vi "GRCtoASPICreg.vi"(1 "TM":bool, 2 "AF1":bool, 3 "RC":u8=3 format="%b", 4 "Gain":u8=8 format="%b") -> (0 "aspic1Data":u32[](array[numeric])=[8388739, 8454144, 8519680, 3722304989, 4008636142, 4294967295, 10, 10, 10, 10, 10, 10, 10, 10, 10, 10, 10, 10, 10, 10, 10, 10, 10, 10, 10, 10, 10, 10, 10, 10, 10, 10] format="%06x")   [LabVIEW 2014]
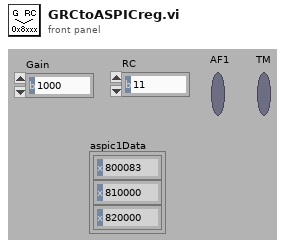
[diagram p1: front panel]
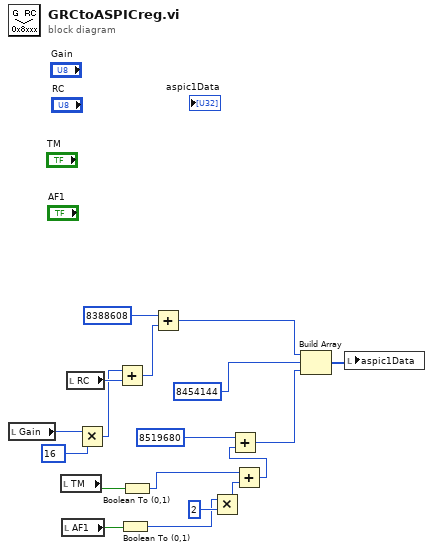
[diagram p0: block diagram]
diagram:
  n1 = local read "Gain"() -> (w14:u8)
  n2 = local read "TM"() -> (w9:bool)
  n3 = local read "AF1"() -> (w10:bool)
  n4 = local read "RC"() -> (w17:u8)
  n5 = Multiply(x=w14, y=u32 16) -> (x*y=w13:u32)
  n6 = Add(x=w13, y=w17) -> (x+y=w16:u32)
  n7 = Boolean To (0,1)(Boolean=w10) -> (0, 1=w7:i16)
  n8 = Boolean To (0,1)(Boolean=w9) -> (0, 1=w6:i16)
  n9 = Add(x=u32 8388608 ("y"), y=w16) -> (x+y=w4:u32)
  n10 = Multiply(x=w7, y=u32 2) -> (x*y=w8:u32)
  n11 = Add(x=w6, y=w8) -> (x+y=w5:u32)
  n12 = Add(x=u32 8519680 ("y"), y=w5) -> (x+y=w2:u32)
  n13 = Build Array(w4, u32 8454144 ("y"), w2) -> (w1:u32[])
  n14 = local write "aspic1Data"(w1) -> ()
